vi "ShortcutMenu.vi"(8 "error in":errorcluster, 9 "menu ref in":refnum<k9>, 11 "CEF_Node in":refnum<class "CEF_Node.lvclass">) -> (0 "error out":errorcluster, 1 "menu ref out":refnum<k9>, 3 "CEF_Node out":refnum<class "CEF_Node.lvclass">)   [LabVIEW 2025, in "CEF.lvlib" / "CEF_Node.lvclass"]
doc: "Defines the behavior of the shortcut menu of the node.Copyright 2017 National Instruments Corporation\n\nLicensed under the Apache License, Version 2.0 (the \"License\"); you may not use this file except in compliance with the License. You may obtain a copy of the License at http://www.apache.org/licenses/LICENSE-2.0\nUnless required by applicable law or agreed to in writing, software distributed under the License is distributed on an \"AS IS\" BASIS, WITHOUT WARRANTIES OR CONDITIONS OF ANY KIND, either express or implied. See the License for the specific language governing permissions and limitations under the License."
uses:
  CEF_Node.lvclass
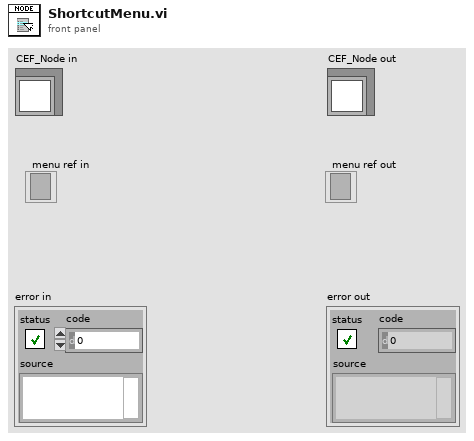
[diagram p1: front panel]
types:
  T1 = typedef "CEF.lvlib/CEF_Node.lvclass/NodeMenuOptions.ctl" = cluster{"removable":bool, "movable":bool, "duplicate":bool}
  T2 = typedef "CEF.lvlib/CEF_Node.lvclass/SubNodeCluster.ctl" = cluster{"subnodes menu name":string[], "subnodes class":string[], "subnodes category":string[]}
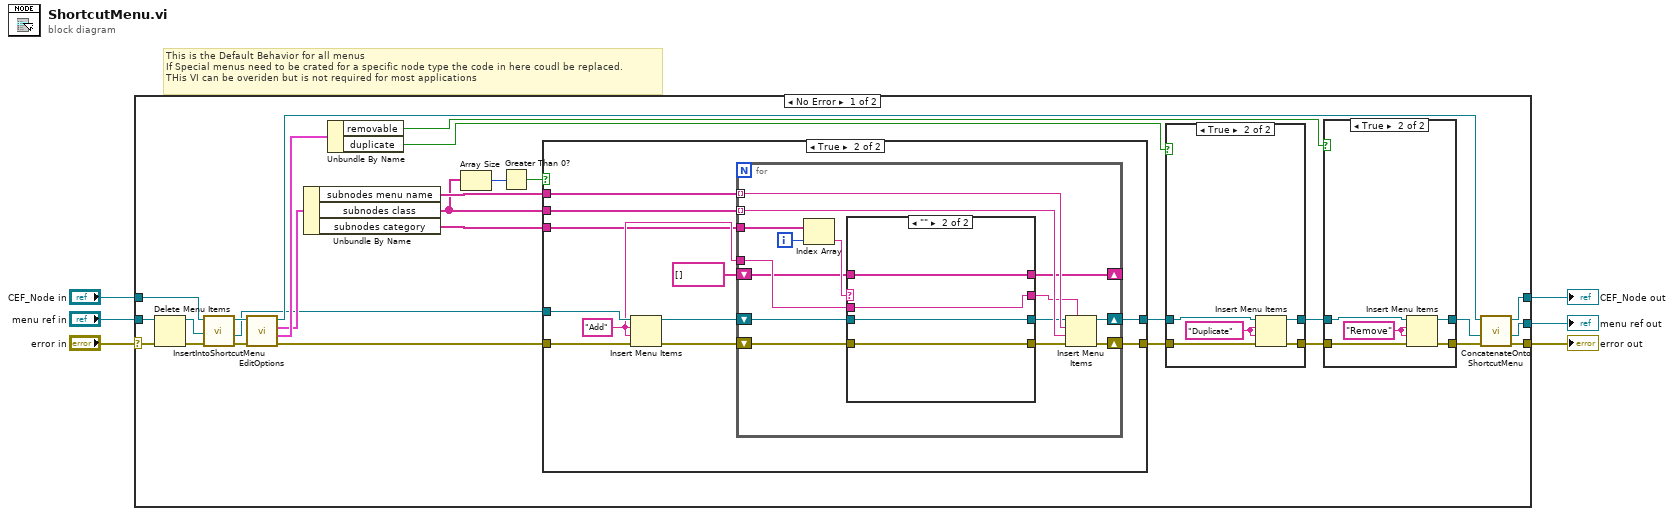
[diagram p0: block diagram]
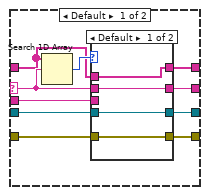
[diagram p5: hidden frame]
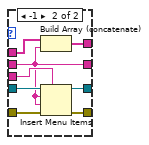
[diagram p6: hidden frame]
diagram:
  # "This is the Default Behavior for all menus\nIf Special menus need to be crated for a specific node type the code in here coudl be replaced.\nTHis VI can be overiden but is not required for most applications"
  n1 = case shown="No Error" "error in" {
    selector: "error in" -> [w27 w104]
    tunnel: [w15 w105] -> w4
    tunnel: "CEF_Node in" -> [w21 w105]
    tunnel: "menu ref in" -> [w30 w103]
    tunnel: [w13 w104] -> w2
    tunnel: [w11 w103] -> w1
    frame No Error {
      n2 = Delete Menu Items(6:w27, 9:w30) -> (0:w19:errorcluster, 3:w7:refnum<k9>)  [unwired: 2 in]
      n3 = call-dynamic "InsertIntoShortcutMenu.vi"("error in"=w19, "menu ref in"=w7, "CEF_Node in"=w21) -> ("error out"=w18:errorcluster, "menu ref out"=w8:refnum<k9>, "CEF_Node out"=w20:refnum<class "CEF_Node.lvclass">)  [unwired: 6 in]
      n4 = call-dynamic "EditOptions.vi"("error in"=w18, "CEF_Node in"=w20) -> ("error out"=w17:errorcluster, "edit options"=w29:T1, "subnodes class"=w10:T2, "CEF_Node out"=w16:refnum<class "CEF_Node.lvclass">)  [unwired: 6 in]
      n5 = Unbundle By Name(w10) -> ("subnodes menu name"=w23:string[], "subnodes class"=w22:string[], "subnodes category"=w9:string[])
      n6 = Unbundle By Name(w29) -> ("removable"=w24:bool, "duplicate"=w28:bool)
      n7 = Array Size(array=w22) -> (size(s)=w34:i32)
      n8 = Greater Than 0?(x=w34) -> (x > 0?=w33:bool)
      n9 = case shown="True" w33 {
        tunnel: w8 -> [w50 w61]
        tunnel: w17 -> [w49 w60]
        tunnel: w23 -> [_ w57]
        tunnel: [w50 w56] -> w32
        tunnel: [w49 w55] -> w31
        tunnel: w22 -> [_ w54]
        tunnel: w9 -> [_ w52]
        frame False {
        }
        frame True {
          w53 = "Add"
          n10 = Insert Menu Items(6:w60, 7:w53, 8:w53, 9:w61) -> (0:w58:errorcluster, 3:w59:refnum<k9>)  [unwired: 2 in, 1 out]
          n11 = for {
            tunnel: w53 -> [w68]
            tunnel: w57 -> [w74] mode=indexing
            shift-right: [w76] -> w56
            shift-left: w59 -> [w65]
            shift-right: [w75] -> w55
            shift-left: w58 -> [w63]
            tunnel: w54 -> [w73] mode=indexing
            tunnel: w52 -> [w72]
            shift-right: [w66] -> _
            shift-left: string[] [] -> [w67]
            i -> [w71]
            n12 = Index Array(array=w72, index=w71) -> (element=w70:string)
            n13 = case shown="\"\"" w70 {
              selector: w70 -> [w84 _]
              tunnel: [w85 w102] -> w69
              tunnel: w68 -> [w79 w102]
              tunnel: w67 -> [w83 w101]
              tunnel: [w82 w101] -> w66
              tunnel: w65 -> [w81 w100]
              tunnel: [w80 w100] -> w64
              tunnel: w63 -> [w78 w99]
              tunnel: [w77 w99] -> w62
              frame Default {
                n14 = Search 1D Array(1D array=w83, element=w84) -> (index of element=w86:i32)  [unwired: 1 in]
                n15 = case shown="Default" w86 {
                  tunnel: [w88 w93] -> w85
                  tunnel: w84 -> [w88 w93]
                  tunnel: w83 -> [w89 w98]
                  tunnel: [w89 w97] -> w82
                  tunnel: w81 -> [w90 w96]
                  tunnel: [w90 w95] -> w80
                  tunnel: w79 -> [_ w94]
                  tunnel: w78 -> [w87 w92]
                  tunnel: [w87 w91] -> w77
                  frame Default {
                  }
                  frame -1 {
                    n16 = Build Array (concatenate)(w98, w93) -> (w97:string[])
                    n17 = Insert Menu Items(5:w94, 6:w92, 7:w93, 8:w93, 9:w96) -> (0:w91:errorcluster, 3:w95:refnum<k9>)  [unwired: 1 in, 1 out]
                  }
                }
              }
              frame "" {
              }
            }
            n18 = Insert Menu Items(5:w69, 6:w62, 7:w73, 8:w74, 9:w64) -> (0:w75:errorcluster, 3:w76:refnum<k9>)  [unwired: 1 in, 1 out]
          }
        }
      }
      n19 = case shown="True" w28 {
        tunnel: w32 -> [w43 w48]
        tunnel: w31 -> [w42 w47]
        tunnel: [w43 w46] -> w25
        tunnel: [w42 w45] -> w26
        frame False {
        }
        frame True {
          w44 = "Duplicate"
          n20 = Insert Menu Items(6:w47, 7:w44, 8:w44, 9:w48) -> (0:w45:errorcluster, 3:w46:refnum<k9>)  [unwired: 2 in, 1 out]
        }
      }
      n21 = case shown="True" w24 {
        tunnel: w26 -> [w36 w41]
        tunnel: [w36 w40] -> w14
        tunnel: w25 -> [w35 w39]
        tunnel: [w35 w38] -> w12
        frame False {
        }
        frame True {
          w37 = "Remove"
          n22 = Insert Menu Items(6:w41, 7:w37, 8:w37, 9:w39) -> (0:w40:errorcluster, 3:w38:refnum<k9>)  [unwired: 2 in, 1 out]
        }
      }
      n23 = call-dynamic "ConcatenateOntoShortcutMenu.vi"("error in"=w14, "menu ref in"=w12, "node in"=w16) -> ("error out"=w13:errorcluster, "menu ref out"=w11:refnum<k9>, "node out"=w15:refnum<class "CEF_Node.lvclass">)  [unwired: 6 in]
    }
    frame Error {
    }
  }
  "error out" <- w2
  "CEF_Node out" <- w4
  "menu ref out" <- w1
